vi "phys_to_img_coords.vi"(5 "fov_y":sgl, 7 "fov_x":sgl, 10 "y":sgl, 11 "x":sgl) -> (2 "image_y":dbl, 3 "image_x":dbl)   [LabVIEW 2023, in "Vision.lvlib"]
uses:
  Vision.lvlib
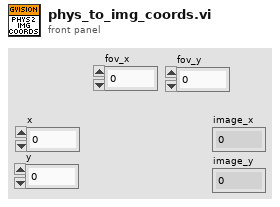
[diagram p1: front panel]
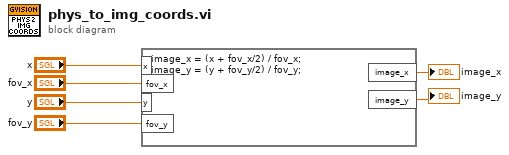
[diagram p0: block diagram]
diagram:
  n1 = formula code="image_x = (x + fov_x/2) / fov_x;\nimage_y = (y + fov_y/2) / fov_y;"("x"="x", "y"="y", "fov_x"="fov_x", "fov_y"="fov_y") -> ("image_x"=→"image_x":dbl, "image_y"=→"image_y":dbl)
